vi "Measure Average WF.vi"(6 "Zernike fit?":bool, 7 "Command":T1, 8 "error in":errorcluster, 11 "Average count":u8=1 min=1 step=1) -> (0 "error out":errorcluster, 2 "WF cluster out":T2)   [LabVIEW 2016]
doc: "This VI reads wavefront measurement from the Thorlabs Shack-Hartmann sensor N times (Average count terminal) and outputs the averaged results.\nThe results of Zernike polynomials fitting are also averaged. \nUnbundle the output cluster for indiviual data arrays."
uses:
  Type definitions/WFS wavefront data.ctl
  Type definitions/States in Measure Average WF.ctl
  Type definitions/State control in WFS_Thorlabs_FGV.ctl
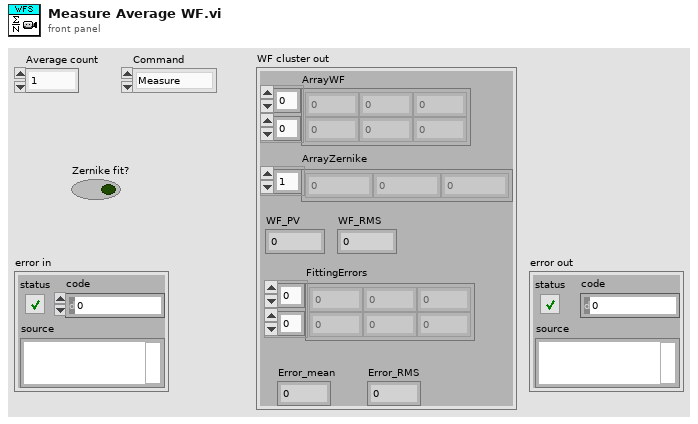
[diagram p1: front panel]
types:
  T1 = typedef "States in Measure Average WF.ctl" = enum16{"Measure", "Read last measurement"}
  T2 = typedef "WFS wavefront data.ctl" = cluster{"ArrayWF":sgl[][], "ArrayZernike":sgl[], "WF_PV":dbl, "WF_RMS":dbl, "FittingErrors":dbl[][], "Error_mean":dbl, "Error_RMS":dbl}
  T3 = typedef "State control in WFS_Thorlabs_FGV.ctl" = enum16{"Initialize", "Configure", "Measure", "Exit"}
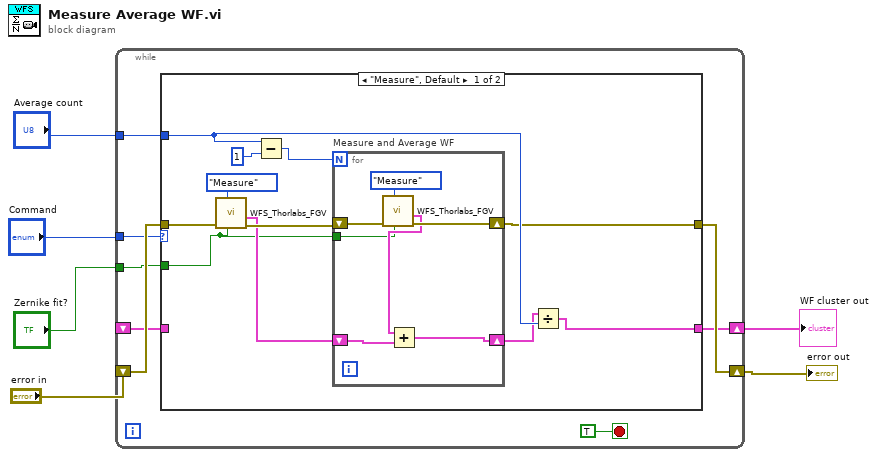
[diagram p0: block diagram]
diagram:
  n1 = while {
    tunnel: "Average count" -> [w14]
    shift-right: [w12] -> w4
    shift-left: "error in" -> [w13]
    shift-right: [w11] -> w3
    shift-left: _ -> [w8]
    tunnel: "Command" -> [w9]
    tunnel: "Zernike fit?" -> [w7]
    stop <- TRUE stop-if-true
    n2 = case shown="\"Measure\", Default" w9 {
      tunnel: w14 -> [w25 _]
      tunnel: w13 -> [w24 w33]
      tunnel: [w23 w33] -> w12
      tunnel: [w22 w34] -> w11
      tunnel: w8 -> [_ w34]
      tunnel: w7 -> [w15 _]
      frame "Measure", Default {
        n3 = call "WFS_Thorlabs_FGV.vi"("Zernike fit?"=w15, "State"=State_control_in_WFS_Thorlabs_FGV."Measure", "error in"=w24) -> ("error out"=w18:errorcluster, "WF data Out"=w16:T2)  [unwired: 6 in, 1 out]
        n4 = Subtract(x=w25, y=u8 1) -> (x-y=w19:u8)
        n5 = for "Measure and Average WF" {
          N: w19 -> [_]
          shift-right: [w30] -> w23
          shift-left: w18 -> [w32]
          shift-right: [w28] -> w21
          shift-left: w16 -> [w29]
          tunnel: w15 -> [w26]
          n6 = call "WFS_Thorlabs_FGV.vi"("Zernike fit?"=w26, "State"=State_control_in_WFS_Thorlabs_FGV."Measure", "error in"=w32) -> ("error out"=w30:errorcluster, "WF data Out"=w27:T2)  [unwired: 6 in, 1 out]
          n7 = Add(x=w27, y=w29) -> (x+y=w28:T2)
        }
        n8 = Divide(x=w21, y=w25) -> (x/y=w22:T2)
      }
      frame "Read last measurement" {
      }
    }
  }
  "error out" <- w4
  "WF cluster out" <- w3
